vi "Producer Consumer Data.vi"() -> ()   [LabVIEW 2012]
doc: "Use this template to build a producer/consumer design pattern. Use this template when you need to execute a process, such as data analysis, when a data source, such as a triggered acquisition, produces data at an uneven rate and you need to execute the process when the data becomes available."
panel:
  out "Queue Backlog":i32(slide) scale=0.0..100.0
  in  "Wait(ms) in Consumer Loop":u32(slide) scale=0.0..10000.0
  out "Dequeued Data":string="element"
  in  "Data to Enqueue":string="element"
  in  "Enqueue Data":bool
  in  "stop":bool
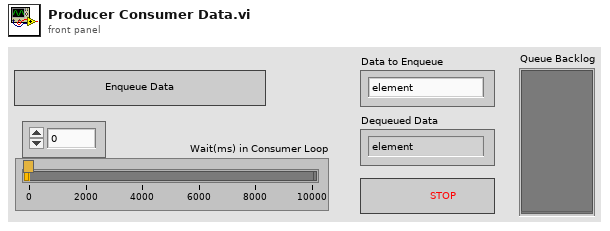
[diagram p1: front panel]
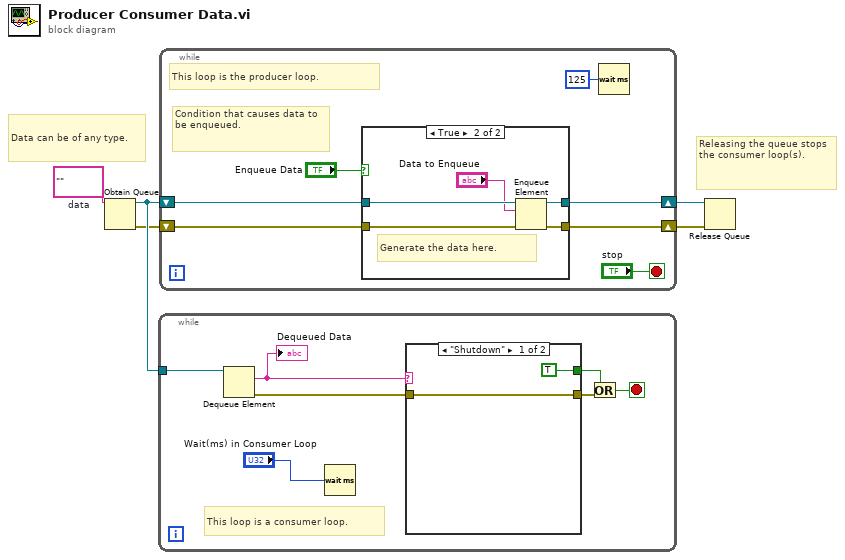
[diagram p0: block diagram]
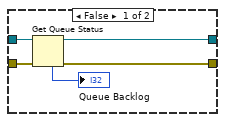
[diagram p3: hidden frame]
diagram:
  w1 = ""  # data
  # "Data can be of any type."
  # "Releasing the queue stops the consumer loop(s)."
  n1 = Obtain Queue(element data type=w1) -> (queue out=w5:refnum<queue>, error out=w4:errorcluster)  [unwired: 4 in, 1 out]
  n2 = while {
    tunnel: w5 -> [w12]
    stop <- w9 stop-if-true
    # "This loop is a consumer loop."
    n3 = Dequeue Element(queue=w12) -> (element=w6:string, error out=w11:errorcluster)  [unwired: 2 in, 2 out]
    "Dequeued Data" <- w6
    n4 = Wait (ms)(milliseconds to wait="Wait(ms) in Consumer Loop") -> ()  [unwired: 1 out]
    n5 = case shown="\"Shutdown\"" w6 {
      tunnel: [TRUE _] -> w8
      tunnel: [w13 w15] -> w10
      tunnel: w11 -> [w13 w15]
      frame "Shutdown" {
      }
      frame Default {
      }
    }
    n6 = Or(x=w8, y=w10) -> (x .or. y?=w9:bool)
  }
  n7 = while {
    shift-right: [w18] -> w2
    shift-left: w4 -> [w19]
    shift-right: [w20] -> w3
    shift-left: w5 -> [w21]
    stop <- "stop" stop-if-true
    # "Condition that causes data to be enqueued."
    # "This loop is the producer loop."
    n8 = case shown="True" "Enqueue Data" {
      tunnel: w21 -> [w25 w32]
      tunnel: [w24 w31] -> w20
      tunnel: w19 -> [w27 w30]
      tunnel: [w26 w29] -> w18
      frame False {
        n9 = Get Queue Status(queue=w25, error in (no error)=w27) -> (queue out=w24:refnum<queue>, error out=w26:errorcluster, # elements in queue=→"Queue Backlog":i32)  [unwired: 1 in, 5 out]
      }
      frame True {
        # "Generate the data here."
        n10 = Enqueue Element(queue=w32, element="Data to Enqueue", error in (no error)=w30) -> (queue out=w31:refnum<queue>, error out=w29:errorcluster)  [unwired: 1 in, 1 out]
      }
    }
    n11 = Wait (ms)(milliseconds to wait=u32 125) -> ()  [unwired: 1 out]
  }
  n12 = Release Queue(queue=w3, error in (no error)=w2) -> ()  [unwired: 1 in, 3 out]
